vi "ModifyMsgIcon.vi"(8 "error in (no error)":errorcluster, 11 "CS++Actor in":refnum<class "CS++Actor.lvclass">) -> (0 "error out":errorcluster, 3 "CS++Actor out":refnum<class "CS++Actor.lvclass">)   [LabVIEW 2015, in "CS++Actor.lvlib" / "CS++Actor.lvclass"]
doc: "This Vi modifies the Icon of the new created message class."
uses:
  CS++Actor.lvclass
  <vilib>/LabVIEW Icon API/API_Text.ctl
  <vilib>/LabVIEW Icon API/lv_icon/Controls/Layer.ctl
  <vilib>/LabVIEW Icon API/lv_icon/Classes/Layer/Layer.lvclass
  <vilib>/LabVIEW Icon API/lv_icon/Controls/LayerType.ctl
  CS++Actor.lvclass/CS++Actor.ctl
  <vilib>/LabVIEW Icon API/lv_icon/Classes/Icon/Icon.lvclass
  <vilib>/LabVIEW Icon API/LabVIEW Icon API.lvlib
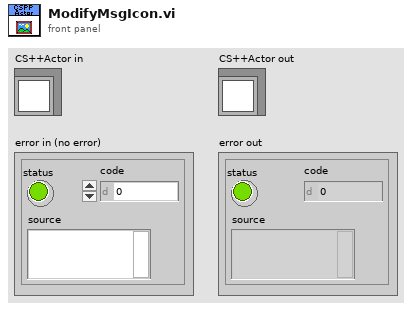
[diagram p1: front panel]
types:
  T1 = typedef "LayerType.ctl" = enum16{"Graphic", "Text", "Tool", "Graphic Drop"}
  T2 = typedef "Layer.ctl" = cluster{"LayerIcon":picture, "LayerName":string, "Opacity":u8, "Visibility?":bool}
  T3 = typedef "LabVIEW Icon API.lvlib/API_Text.ctl" = cluster{"Line 1 text":string, "Line 2 text":string, "Line 3 text":string, "Line 4 text":string}
  T4 = typedef "imagedata.ctl" = cluster{"image type":i32, "image depth":i32, "image":u8[], "mask":u8[], "colors":u32[], "Rectangle":cluster{"left":i16, "top":i16, "right":i16, "bottom":i16}}
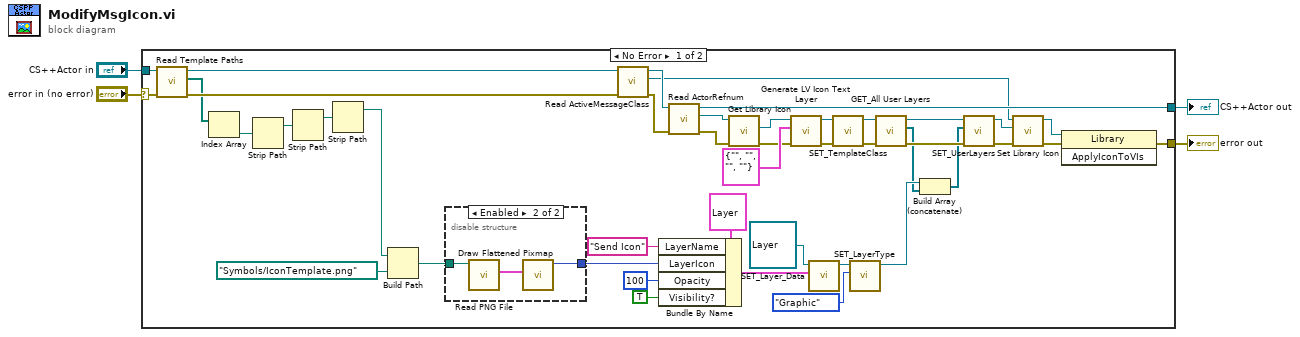
[diagram p0: block diagram]
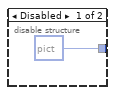
[diagram p2: hidden frame]
diagram:
  n1 = case shown="No Error" "error in (no error)" {
    selector: "error in (no error)" -> [w13 w53]
    tunnel: [w47 w53] -> w3
    tunnel: [w45 w52] -> w1
    tunnel: "CS++Actor in" -> [w15 w52]
    frame No Error {
      n2 = call "Read Template Paths.vi"("error in (no error)"=w13, "CS++Actor in"=w15) -> ("error out"=w12:errorcluster, "Template Paths"=w6:path[], "CS++Actor out"=w14:refnum<class "CS++Actor.lvclass">)  [unwired: 7 in]
      n3 = Index Array(array=w6) -> (element=w5:path)  [unwired: 1 in]
      n4 = Strip Path(path=w5) -> (stripped path=w11:path)  [unwired: 1 out]
      n5 = Strip Path(path=w11) -> (stripped path=w10:path)  [unwired: 1 out]
      n6 = Strip Path(path=w10) -> (stripped path=w9:path)  [unwired: 1 out]
      n7 = Build Path(base path=w9, name or relative path=path "Symbols/IconTemplate.png" ("path to PNG file")) -> (appended path=w7:path)
      n8 = disable-structure shown="Enabled" {
        disable-tunnel: [picture bytes[1182] ("new picture 2") w50] -> w18
        disable-tunnel: w7 -> [_ w49]
        frame Disabled {
        }
        frame Enabled {
          n9 = call <vilib>:"Read PNG File.vi"("path to PNG file"=w49) -> ("image data"=w51:T4)  [unwired: 8 in, 2 out]
          n10 = call <vilib>:"Draw Flattened Pixmap.vi"("image data"=w51) -> ("new picture"=w50:picture)  [unwired: 8 in]
        }
      }
      n11 = call "Read ActiveMessageClass.vi"("error in (no error)"=w12, "CS++Actor in"=w14) -> ("error out"=w44:errorcluster, "ActiveMessageClass"=w30:refnum<vi>, "CS++Actor out"=w46:refnum<class "CS++Actor.lvclass">)  [unwired: 7 in]
      n12 = Bundle By Name(cluster=T2 {"LayerIcon"=bytes[3102], "LayerName"="", "Opacity"=100, "Visibility?"=TRUE} ("Data"), "LayerName"="Send Icon", "LayerIcon"=w18, "Opacity"=u8 100, "Visibility?"=TRUE) -> (w24:T2)
      n13 = call "Read ActorRefnum.vi"("error in (no error)"=w44, "CS++Actor in"=w46) -> ("error out"=w42:errorcluster, "ActorRefnum"=w43:refnum<vi>, "CS++Actor out"=w45:refnum<class "CS++Actor.lvclass">)  [unwired: 7 in]
      n14 = call <vilib>:"Get Library Icon.vi"("error in (no error)"=w42, "Library Refnum in"=w43) -> ("error out"=w34:errorcluster, "Icon"=w33:refnum<class "Icon.lvclass">)  [unwired: 7 in, 1 out]
      n15 = call <vilib>:"Generate LV Icon Text Layer.vi"("error in (no error)"=w34, "Text"=T3 {"Line 1 text"="", "Line 2 text"="", "Line 3 text"="", "Line 4 text"=""}, "Icon in"=w33) -> ("error out"=w40:errorcluster, "Icon out"=w38:refnum<class "Icon.lvclass">)  [unwired: 7 in]
      n16 = call-dynamic "SET_Layer_Data.vi"("Data"=w24, "Layer.lvclass in"=refnum<class "Layer.lvclass"> refnum) -> ("Layer.lvclass out"=w26:refnum<class "Layer.lvclass">)  [unwired: 2 in, 7 out]
      n17 = call-dynamic "SET_TemplateClass.vi"("error in (no error)"=w40, "Icon.lvclass in"=w38) -> ("error out"=w39:errorcluster, "Icon.lvclass out"=w37:refnum<class "Icon.lvclass">)  [unwired: 8 in]
      n18 = call-dynamic "SET_LayerType.vi"("Type"=LayerType."Graphic", "Layer.lvclass in"=w26) -> ("Layer.lvclass out"=w25:refnum<class "Layer.lvclass">)  [unwired: 1 in, 8 out]
      n19 = call-dynamic "GET_All User Layers.vi"("error in (no error)"=w39, "Icon.lvclass in"=w37) -> ("error out"=w35:errorcluster, "User Layer"=w17:refnum<class "Layer.lvclass">[], "Icon.lvclass out"=w36:refnum<class "Icon.lvclass">)  [unwired: 7 in]
      n20 = Build Array (concatenate)(w25, w17) -> (w16:refnum<class "Layer.lvclass">[])
      n21 = call-dynamic "SET_UserLayers.vi"("error in (no error)"=w35, "Layers"=w16, "Icon.lvclass in"=w36) -> ("error out"=w32:errorcluster, "Icon.lvclass out"=w28:refnum<class "Icon.lvclass">)  [unwired: 7 in]
      n22 = call <vilib>:"Set Library Icon.vi"("error in (no error)"=w32, "Icon"=w28, "Library Refnum in"=w30) -> ("error out"=w31:errorcluster, "Library Refnum out"=w29:refnum<vi>)  [unwired: 7 in]
      n23 = invoke class="Library" method="ApplyIconToVIs"(reference=w29, error in=w31) -> (error out=w47:errorcluster)  [unwired: 1 in, 2 out]
    }
    frame Error {
    }
  }
  "error out" <- w3
  "CS++Actor out" <- w1
